vi "Sensor mode test.vi"() -> ()   [LabVIEW 2017]
uses:
  C:/Program Files/National Instruments/LabVIEW 2017/instr.lib/IDS/ueye.NET/uEyeDotNet.dll
panel:
  in  "reference":refnum<k24>
  in  "mode in":i32(ring) items=["BGRA8Packed"=0, "BGR8Packed"=1, "BGR565Packed"=2, "BGR5Packed"=3, "Mono8"=6, "SensorRaw8"=11, "UYVYPacked"=12, "UYVYMonoPacked"=13, "UYVYBayerPacked"=14, "CBYCRYPacked"=23, "BGRY8Packed"=24, "BGR10Packed"=25, "Mono12"=26, "SensorRaw12"=27, "Mono16"=28, "SensorRaw16"=29, "BGR12Unpacked"=30, "BGRA12Unpacked"=31, "Jpeg"=32, "BGR10Unpacked"=35, "RGBA8Packed"=128, "RGB8Packed"=129, "RGBY8Packed"=152, "RGB10Packed"=153, "RGB12Unpacked"=158, "RGBA12Unpacked"=159, "RGB10Unpacked"=163, "RGB8Planar"=8321, "PreferPackedSourceFormat"=16384]
  out "Numeric mode":i32
  out "mode out":i32(ring) items=["BGRA8Packed"=0, "BGR8Packed"=1, "BGR565Packed"=2, "BGR5Packed"=3, "Mono8"=6, "SensorRaw8"=11, "UYVYPacked"=12, "UYVYMonoPacked"=13, "UYVYBayerPacked"=14, "CBYCRYPacked"=23, "BGRY8Packed"=24, "BGR10Packed"=25, "Mono12"=26, "SensorRaw12"=27, "Mono16"=28, "SensorRaw16"=29, "BGR12Unpacked"=30, "BGRA12Unpacked"=31, "Jpeg"=32, "BGR10Unpacked"=35, "RGBA8Packed"=128, "RGB8Packed"=129, "RGBY8Packed"=152, "RGB10Packed"=153, "RGB12Unpacked"=158, "RGBA12Unpacked"=159, "RGB10Unpacked"=163, "RGB8Planar"=8321, "PreferPackedSourceFormat"=16384]
  out "SensorColorMode":i32(ring) items=["Invalid"=0, "Monochrome"=1, "Bayer"=2, "CBYCRY"=4, "Jpeg"=8]
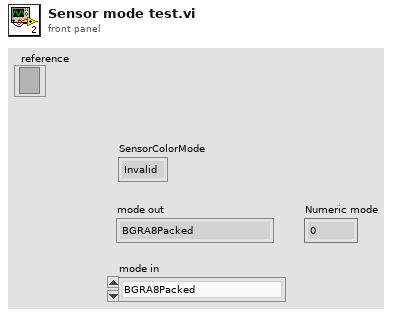
[diagram p1: front panel]
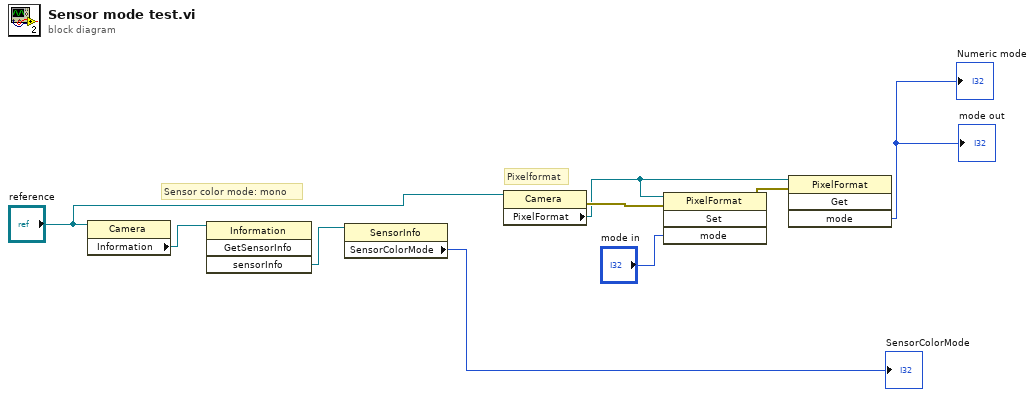
[diagram p0: block diagram]
diagram:
  # "Pixelformat"
  # "Sensor color mode: mono"
  n1 = property on="Eigenschaftsknoten" class="Camera"(reference="reference") -> ("Information"=w9:refnum<k24>)  [unwired: 1 in, 2 out]
  n2 = invoke class="Information" method="GetSensorInfo"(reference=w9) -> ("sensorInfo"=w8:refnum<k24>)  [unwired: 3 in, 3 out]
  n3 = property class="SensorInfo"(reference=w8) -> ("SensorColorMode"=→"SensorColorMode":i32)  [unwired: 1 in, 2 out]
  n4 = property class="Camera"(reference="reference") -> (error out=w5:errorcluster, "PixelFormat"=w3:refnum<k24>)  [unwired: 1 in, 1 out]
  n5 = invoke class="PixelFormat" method="Set"(reference=w3, error in=w5, "mode"="mode in") -> (error out=w4:errorcluster)  [unwired: 1 in, 3 out]
  n6 = invoke class="PixelFormat" method="Get"(reference=w3, error in=w4) -> ("mode"=→"mode out" →"Numeric mode":i32)  [unwired: 2 in, 3 out]
